vi "Export Data to TDMS.vi"(11 "WaveformGraph in":refnum<vi>) -> (0 "error out":errorcluster)   [LabVIEW 2025, in "Ni-Scope-Multirecords UI.lvlib"]
uses:
  Ni-Scope-Multirecords UI.lvlib
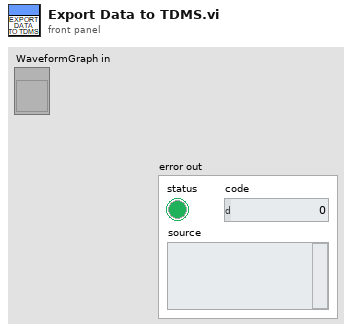
[diagram p1: front panel]
types:
  T1 = cluster{"relativeInitialX":dbl, "xIncrement":dbl, "wfm":dbl[]}[]
  T2 = enum16{"open", "open or create", "create or replace", "create", "open (read-only)"}
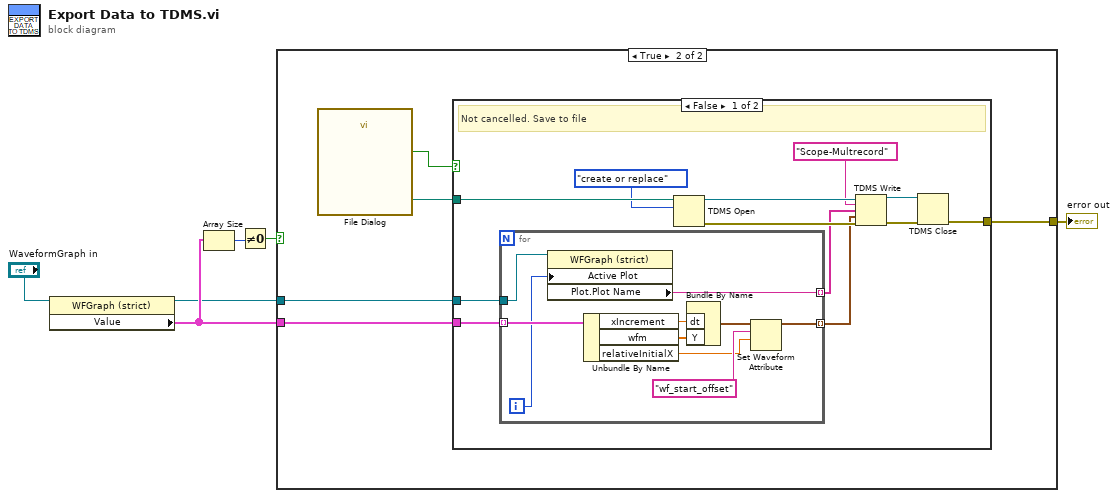
[diagram p0: block diagram]
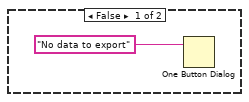
[diagram p2: hidden frame]
diagram:
  n1 = property class="WFGraph (strict)"(reference="WaveformGraph in") -> (reference out=w2:refnum<vi>, "Value"=w5:T1)  [unwired: 1 in, 1 out]
  n2 = Array Size(array=w5) -> (size(s)=w4:i32)
  n3 = Not Equal To 0?(x=w4) -> (x != 0?=w3:bool)
  n4 = case shown="True" w3 {
    tunnel: w5 -> [_ w12]
    tunnel: w2 -> [_ w9]
    tunnel: [_ w8] -> w1
    frame False {
      n5 = One Button Dialog(message="No data to export") -> ()  [unwired: 1 in, 1 out]
    }
    frame True {
      n6 = call "File Dialog"() -> ("selected path"=w11:path, "cancelled"=w10:bool)  [unwired: 12 in, 2 out]
      n7 = case shown="False" w10 {
        tunnel: w11 -> [w24 _]
        tunnel: w12 -> [w19 _]
        tunnel: w9 -> [w18 _]
        tunnel: [w13 _] -> w8
        frame False {
          # "Not cancelled. Save to file"
          n8 = for {
            tunnel: w19 -> [w34] mode=indexing
            tunnel: w18 -> [w31]
            tunnel: [w29] -> w17 mode=indexing
            tunnel: [w27] -> w16 mode=indexing
            i -> [w30]
            n9 = property class="WFGraph (strict)"(reference=w31, "Active Plot"=w30) -> ("Plot.Plot Name"=w29:string)  [unwired: 1 in, 2 out]
            n10 = Unbundle By Name(w34) -> ("xIncrement"=w32:dbl, "wfm"=w33:dbl[], "relativeInitialX"=w25:dbl)
            n11 = Bundle By Name("dt"=w32, "Y"=w33) -> (w28:waveform(dbl))  [unwired: 1 in]
            n12 = Set Waveform Attribute(5:w25, 6:"wf_start_offset" ("name"), 7:w28) -> (3:w27:waveform(dbl))  [unwired: 1 in, 2 out]
          }
          n13 = TDMS Open(10:T2."create or replace" ("operation (0:open)"), 11:w24) -> (0:w21:errorcluster, 3:w22:refnum<k34>)  [unwired: 5 in]
          n14 = TDMS Write(0:w22, 5:"Scope-Multrecord" ("group name in (Untitled)"), 7:w17, 9:w16, 11:w21) -> (4:w15:refnum<k34>, 15:w14:errorcluster)  [unwired: 1 in, 2 out]
          n15 = TDMS Close(8:w14, 11:w15) -> (0:w13:errorcluster)  [unwired: 1 out]
        }
        frame True {
        }
      }
    }
  }
  "error out" <- w1
